vi "AFT Linear Prediction (PtbyPt).vi"(6 "step size":dbl=-1.0, 7 "reset? (F)":bool, 8 "error in (no error)":errorcluster, 10 "signal":dbl, 11 "adaptive filter in":refnum<k20>) -> (0 "error out":errorcluster, 1 "prediction error":dbl, 3 "adaptive filter out":refnum<k20>, 4 "AR coefficients":dbl[](array[numeric]))   [LabVIEW 2017, in "NI_AdaptiveFilter.lvlib"]
doc: "Performs adaptive linear prediction by estimating the autoregressive (AR) model of an input signal. Wire data to the <B>signal</B> input to determine the polymorphic instance to use or manually select the instance."
uses:
  <vilib>/addons/Adaptive Filters/NI_AdaptiveFilter.lvlib
  <vilib>/addons/Adaptive Filters/Analysis/AFT Get Coefficients (FIR, Real).vi
  <vilib>/addons/Adaptive Filters/Processing/AFT Filter Signal and Update Coefficients (Real, PtByPt).vi
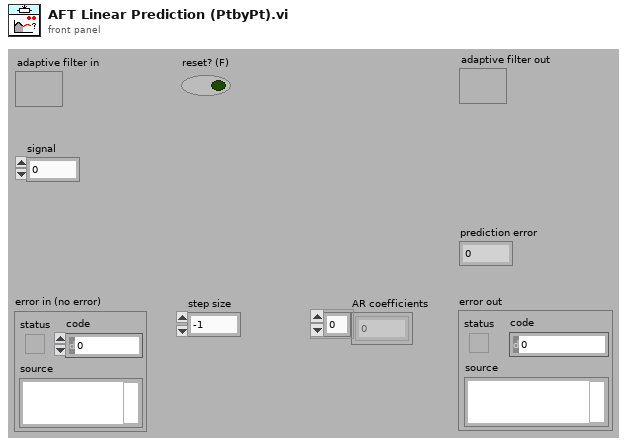
[diagram p1: front panel]
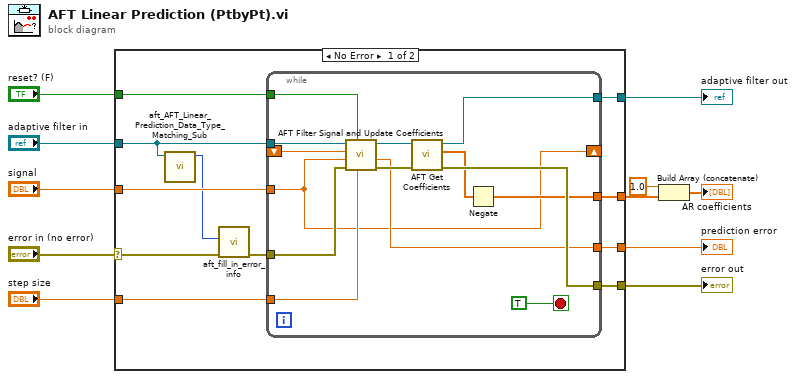
[diagram p0: block diagram]
diagram:
  n1 = case shown="No Error" "error in (no error)" {
    selector: "error in (no error)" -> [w14 w38]
    tunnel: "adaptive filter in" -> [w12 w37]
    tunnel: [w22 w37] -> w10
    tunnel: "signal" -> [w21 _]
    tunnel: [w20 w38] -> w7
    tunnel: "reset? (F)" -> [w19 _]
    tunnel: "step size" -> [w18 _]
    tunnel: [w17 _] -> w1
    tunnel: [w16 _] -> w4
    frame No Error {
      n2 = call <vilib>:"aft_AFT_Linear_Prediction_Data_Type_Matching_Sub.vi"("adaptive filter in"=w12) -> ("error"=w15:i32)  [unwired: 10 out]
      n3 = call <vilib>:"aft_fill_in_error_info.vi"("error in"=w14, "status code"=w15) -> ("error out"=w13:errorcluster)  [unwired: 2 in, 7 out]
      n4 = while {
        tunnel: w12 -> [w36]
        tunnel: [w29] -> w22
        shift-right: [w23] -> _
        shift-left: _ -> [w24]
        tunnel: w21 -> [w23]
        tunnel: w13 -> [w35]
        tunnel: [w30] -> w20
        tunnel: w19 -> [w34]
        tunnel: w18 -> [w33]
        tunnel: [w25] -> w17
        tunnel: [w26] -> w16
        stop <- TRUE stop-if-true
        n5 = call-poly <vilib>:"AFT Filter Signal and Update Coefficients.vi"("step size"=w33, "reset? (F)"=w34, "error in (no error)"=w35, "d(n)"=w23, "x(n)"=w24, "adaptive filter in"=w36) -> ("error out"=w31:errorcluster, "e(n)"=w26:dbl, "adaptive filter out"=w32:refnum<k20>)  [unwired: 3 out]
        n6 = call-poly <vilib>:"AFT Get Coefficients.vi"("error in (no error)"=w31, "adaptive filter in"=w32) -> ("error out"=w30:errorcluster, "coefficients"=w28:dbl[], "adaptive filter out"=w29:refnum<k20>)  [unwired: 7 out]
        n7 = Negate(x=w28) -> (-x=w25:dbl[])
      }
    }
    frame Error {
    }
  }
  "adaptive filter out" <- w10
  "error out" <- w7
  "prediction error" <- w4
  n8 = Build Array (concatenate)(1.0 ("element"), w1) -> (→"AR coefficients":dbl[])
